vi "Memory Benchmark.vi"(5 "Show Cache Lines (T)":bool=TRUE, 7 "Show Peak Bandwidth (T)":bool=TRUE, 9 "Transfers (500)":i32=500, 10 "End Size (100MB)":u64=100000000 format="%.0pB", 11 "Start Size (1kB)":u64=1000 format="%.0pB") -> (3 "Memory Bandwidth":cluster{"X":dbl[], "Y":dbl[]}[](graph) caption="Memory Bandwidth Plot")   [LabVIEW 2016]
uses:
  Source/Library/Classes/Pointer/Pointer.Void/Memory.Pointer.Void.lvclass/Memory.Pointer.Void.ctl
  Source/Library/Classes/Pointer/Pointer.Void/Methods/Memory.Pointer.Offset to Address.Unsafe.vi
  Source/Library/Classes/Pointer/Pointer.Void/Methods/Memory.Pointer.Allocate.vi
  Source/Library/Classes/Pointer/Pointer.Void/Methods/Memory.Pointer.Get Address.vi
  Source/Library/Classes/Pointer/Pointer.Void/Methods/Memory.Pointer.Set Address.vi
  Source/Library/Classes/Pointer/Pointer.Void/Methods/Memory.Pointer.Set Size.vi
  Source/Library/Classes/Pointer/Pointer.Void/Memory.Pointer.Void.lvclass
panel:
  out "Peak Throughput":dbl format="%.3pB/s"
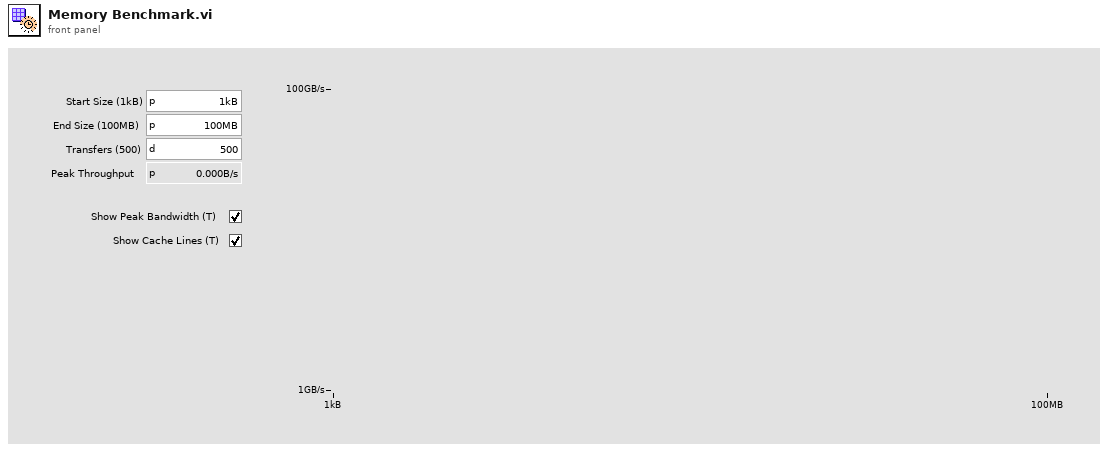
[diagram p1: front panel]
types:
  T1 = typedef "LVAnnotationListTypeDef.ctl" = cluster{"Name":string, "Color":u32, "Style":u8, "Point Style":u8, "Name Visible":bool, "Allow Drag":bool, "Annotation Mode":u32, "Plot":i32, "Index":i32, "Position":cluster{"X":dbl, "Y":dbl}, "X Scale":u32, "Y Scale":u32, "Show Arrow":bool, "Lock Name":bool, "Plot Area":i32, "Label Offset":cluster{"X":dbl, "Y":dbl}}[]
  T2 = cluster{"Name":string, "Color":u32, "Style":u8, "Point Style":u8, "Name Visible":bool, "Allow Drag":bool, "Annotation Mode":u32, "Plot":i32, "Index":i32, "Position":cluster{"X":dbl, "Y":dbl}, "X Scale":u32, "Y Scale":u32, "Show Arrow":bool, "Lock Name":bool, "Plot Area":i32, "Label Offset":cluster{"X":dbl, "Y":dbl}}
  T3 = cluster{"Name":string, "Color":u32, "Style":u8, "Point Style":u8, "Name Visible":bool, "Allow Drag":bool, "Annotation Mode":u32, "Plot":i32, "Index":i32, "Position":cluster{"X":dbl, "Y":dbl}, "X Scale":u32, "Y Scale":u32, "Show Arrow":bool, "Lock Name":bool, "Plot Area":i32, "Label Offset":cluster{"X":dbl, "Y":dbl}}[]
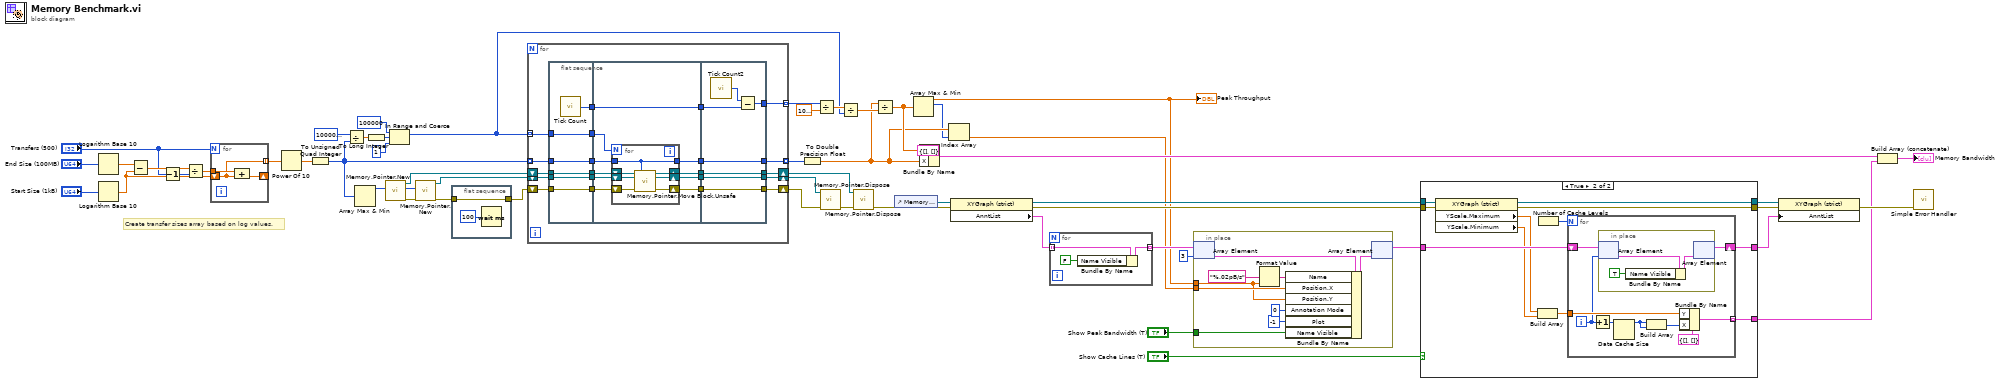
[diagram p0: block diagram]
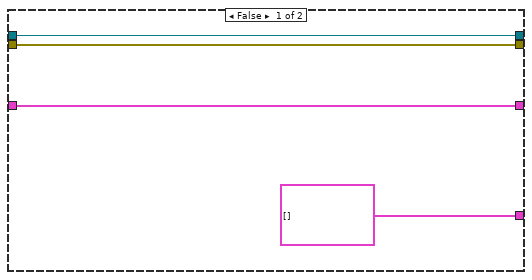
[diagram p2: hidden frame]
diagram:
  # "Create transfer sizes array based on log values."
  n1 = Logarithm Base 10(1:"End Size (100MB)") -> (0:w54:dbl)
  n2 = Logarithm Base 10(1:"Start Size (1kB)") -> (0:w51:dbl)
  n3 = Subtract(x=w54, y=w51) -> (x-y=w53:dbl)
  n4 = Decrement(x="Transfers (500)") -> (x-1=w49:i32)
  n5 = Divide(x=w53, y=w49) -> (x/y=w52:dbl)
  n6 = for {
    N: "Transfers (500)" -> [_]
    tunnel: w52 -> [w59]
    shift-right: [w58] -> _
    shift-left: w51 -> [w57]
    tunnel: [w57] -> w48 mode=indexing
    n7 = Compound Arithmetic op=ADD(w59, w57) -> (w58:dbl)
  }
  n8 = Power Of 10(x=w48) -> (10^x=w47:dbl[])
  n9 = To Unsigned Quad Integer(1:w47) -> (0:w41:u64[])
  n10 = Divide(x=u64 100000000, y=w41) -> (x/y=w40:dbl[])
  n11 = Array Max & Min(array=w41) -> (max value=w29:u64)  [unwired: 3 out]
  n12 = To Long Integer(number=w40) -> (32bit integer=w39:i32[])
  n13 = call "Memory.Pointer.New.vi"("size"=w29) -> ("error out"=w35:errorcluster, "allocated size"=w26:u64, "Pointer out"=w23:refnum<class "Memory.Pointer.Void.lvclass">)  [unwired: 8 in]
  n14 = In Range and Coerce(upper limit=100000, x=w39, lower limit=1) -> (coerced(x)=w16:i32[])  [unwired: 1 out]
  n15 = call "Memory.Pointer.New.vi"("error in (no error)"=w35, "size"=w26) -> ("error out"=w22:errorcluster, "Pointer out"=w36:refnum<class "Memory.Pointer.Void.lvclass">)  [unwired: 7 in, 1 out]
  n16 = flat-sequence {
    tunnel: w22 -> [w61]
    tunnel: [w61] -> w21
    frame #0 {
      n17 = Wait (ms)(milliseconds to wait=u32 100) -> ()  [unwired: 1 out]
    }
  }
  n18 = for {
    shift-right: [w66] -> w33
    shift-left: w36 -> [w70]
    shift-right: [w65] -> w31
    shift-left: w23 -> [w69]
    shift-right: [w67] -> w34
    shift-left: w21 -> [w68]
    tunnel: [w64] -> w28 mode=indexing
    tunnel: w41 -> [w63] mode=indexing
    tunnel: [w62] -> w24 mode=indexing
    tunnel: w16 -> [w71] mode=indexing
    n19 = flat-sequence {
      tunnel: [w88] -> w82
      tunnel: [w87] -> w81
      tunnel: [w86] -> w80
      tunnel: [w85] -> w79
      tunnel: [w84] -> w78
      tunnel: [w83] -> w77
      tunnel: w69 -> [w88]
      tunnel: w70 -> [w87]
      tunnel: w68 -> [w86]
      tunnel: w63 -> [w85]
      tunnel: w71 -> [w84]
      tunnel: w82 -> [w98]
      tunnel: w81 -> [w97]
      tunnel: w80 -> [w96]
      tunnel: w79 -> [w95]
      tunnel: w78 -> [w91]
      tunnel: w77 -> [w90]
      tunnel: [w90] -> w76
      tunnel: [w94] -> w75
      tunnel: [w93] -> w74
      tunnel: [w92] -> w73
      tunnel: [w89] -> w72
      tunnel: w76 -> [w111]
      tunnel: w75 -> [w110]
      tunnel: w74 -> [w109]
      tunnel: w73 -> [w108]
      tunnel: w72 -> [w107]
      tunnel: [w110] -> w67
      tunnel: [w109] -> w65
      tunnel: [w108] -> w66
      tunnel: [w107] -> w62
      tunnel: [w106] -> w64
      frame #0 {
        n20 = call "Tick Count"() -> ("Tick Count(uSec)"=w83:u32)
      }
      frame #1 {
        n21 = for {
          N: w91 -> [_]
          shift-right: [w102] -> w94
          shift-left: w96 -> [w103]
          shift-right: [w101] -> w93
          shift-left: w98 -> [w105]
          shift-right: [w100] -> w92
          shift-left: w97 -> [w104]
          tunnel: w95 -> [w99]
          tunnel: [w99] -> w89
          n22 = call "Memory.Pointer.Move Block.Unsafe.vi"("src Pointer in"=w105, "length"=w99, "dst Pointer in"=w104, "error in (no error)"=w103) -> ("src Pointer out"=w101:refnum<class "Memory.Pointer.Void.lvclass">, "dst Pointer out"=w100:refnum<class "Memory.Pointer.Void.lvclass">, "error out"=w102:errorcluster)  [unwired: 9 in]
        }
      }
      frame #2 {
        n23 = call "Tick Count2"() -> ("Tick Count(uSec)"=w112:u32)
        n24 = Subtract(x=w112, y=w111) -> (x-y=w106:u32)
      }
    }
  }
  n25 = To Double Precision Float(number=w24) -> (double precision float=w20:dbl[])
  n26 = Divide(x=w28, y=1000000.0) -> (x/y=w27:dbl[])
  n27 = call "Memory.Pointer.Dispose.vi"("error in (no error)"=w34, "Pointer in"=w33) -> ("error out"=w32:errorcluster)  [unwired: 9 in]
  n28 = Divide(x=w27, y=w16) -> (x/y=w25:dbl[])
  n29 = call "Memory.Pointer.Dispose.vi"("error in (no error)"=w32, "Pointer in"=w31) -> ("error out"=w6:errorcluster)  [unwired: 9 in]
  n30 = Divide(x=w20, y=w25) -> (x/y=w46:dbl[])
  n31 = control-ref of="Memory Bandwidth"() -> (w14:refnum<vi>)
  n32 = Array Max & Min(array=w46) -> (max value=w8:dbl, max index (indices)=w18:i32)  [unwired: 2 out]
  "Peak Throughput" <- w8
  n33 = Bundle By Name(cluster=cluster{"X":dbl[], "Y":dbl[]} {"X"=[], "Y"=[]}, "Y"=w46, "X"=w20) -> (w44:cluster{"X":dbl[], "Y":dbl[]})
  n34 = Index Array(array=w20, index=w18) -> (element=w7:dbl)
  n35 = property class="XYGraph (strict)"(reference=w14, error in=w6) -> (reference out=w9:refnum<vi>, error out=w10:errorcluster, "AnntList"=w13:T1)
  n36 = for {
    tunnel: w13 -> [w114] mode=indexing
    tunnel: [w113] -> w11 mode=indexing
    n37 = Bundle By Name(cluster=w114, "Name Visible"=FALSE) -> (w113:T2)
  }
  n38 = in-place {
    in-place-border: w8 -> [w116]
    in-place-border: w7 -> [w120]
    in-place-border: "Show Peak Bandwidth (T)" -> [w117]
    n39 = in-place-array #1(w11, 3) -> (w124:T2)
    n40 = Format Value(format string="%.02pB/s", value (0)=w116) -> (output string=w122:string)  [unwired: 1 in]
    n41 = Bundle By Name(cluster=w124, "Name"=w122, "Position.X"=w120, "Position.Y"=w116, "Annotation Mode"=u32 0, "Plot"=-1, "Name Visible"=w117) -> (w121:T2)
    n42 = in-place-array #1(w121) -> (w15:T3)  [unwired: 1 out]
  }
  n43 = case shown="True" "Show Cache Lines (T)" {
    tunnel: [cluster{"X":dbl[], "Y":dbl[]}[] [] w137] -> w1
    tunnel: w9 -> [w125 w136]
    tunnel: w15 -> [w126 w135]
    tunnel: w10 -> [w127 w134]
    tunnel: [w127 w131] -> w5
    tunnel: [w125 w130] -> w4
    tunnel: [w126 w129] -> w3
    frame False {
    }
    frame True {
      n44 = property class="XYGraph (strict)"(reference=w136, error in=w134) -> (reference out=w130:refnum<vi>, error out=w131:errorcluster, "YScale.Maximum"=w133:dbl, "YScale.Minimum"=w132:dbl)
      n45 = Build Array(w133, w132) -> (w138:dbl[])
      n46 = Number of Cache Levels() -> (w139:i32)
      n47 = for {
        N: w139 -> [_]
        tunnel: w138 -> [w144]
        tunnel: [w143] -> w137 mode=indexing
        shift-right: [w141] -> w129
        shift-left: w135 -> [w142]
        i -> [w140]
        n48 = Increment(x=w140) -> (x+1=w148:i32)
        n49 = in-place {
          n50 = in-place-array #2(w142, w140) -> (w151:T2)
          n51 = Bundle By Name(cluster=w151, "Name Visible"=TRUE) -> (w150:T2)
          n52 = in-place-array #2(w150) -> (w141:T3)  [unwired: 1 out]
        }
        n53 = Data Cache Size(0:w148) -> (4:w146:i32)  [unwired: 1 out]
        n54 = Build Array(w146, w146) -> (w145:i32[])
        n55 = Bundle By Name(cluster=cluster{"X":dbl[], "Y":dbl[]} {"X"=[], "Y"=[]}, "Y"=w144, "X"=w145) -> (w143:cluster{"X":dbl[], "Y":dbl[]})
      }
    }
  }
  n56 = property class="XYGraph (strict)"(reference=w4, error in=w5, "AnntList"=w3) -> (error out=w2:errorcluster)  [unwired: 1 out]
  n57 = Build Array (concatenate)(w44, w1) -> (→"Memory Bandwidth":cluster{"X":dbl[], "Y":dbl[]}[])
  n58 = call <vilib>:"Simple Error Handler.vi"("error in (no error)"=w2) -> ()  [unwired: 4 in, 5 out]
